vi "path array.vi"(10 "Array":string[](array[string]), 11 "file path (dialog if empty)":path=path "D:/Gantry_General/Main/ms_kao/gantry path/path data/20211103xxx.TXT") -> (3 "path array":path[](array[path]))   [LabVIEW 2016]
panel:
  out "size(s)":i32
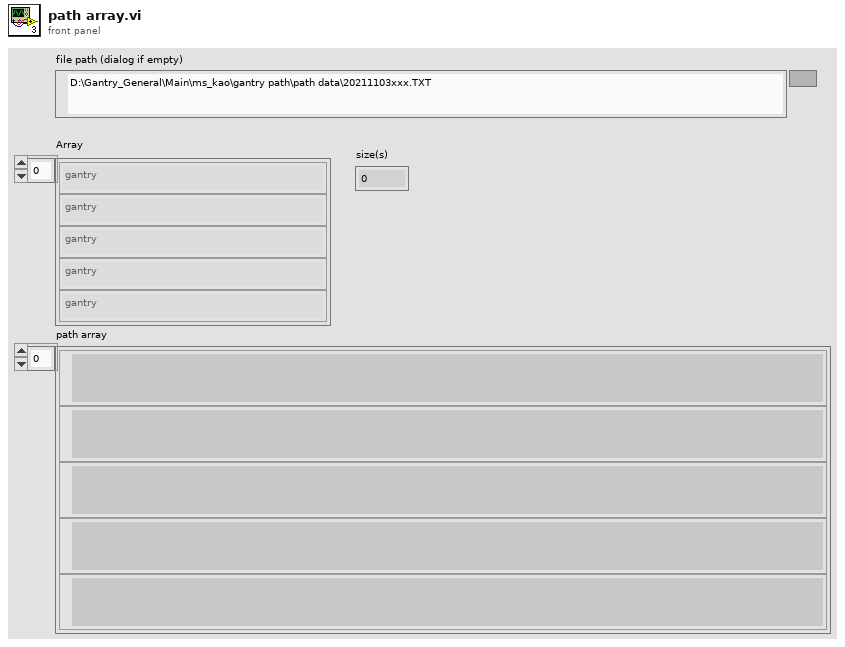
[diagram p1: front panel]
types:
  T1 = cluster{"Path":path, "folder name":string, "file name":string, "extension":string, "add time string":bool}
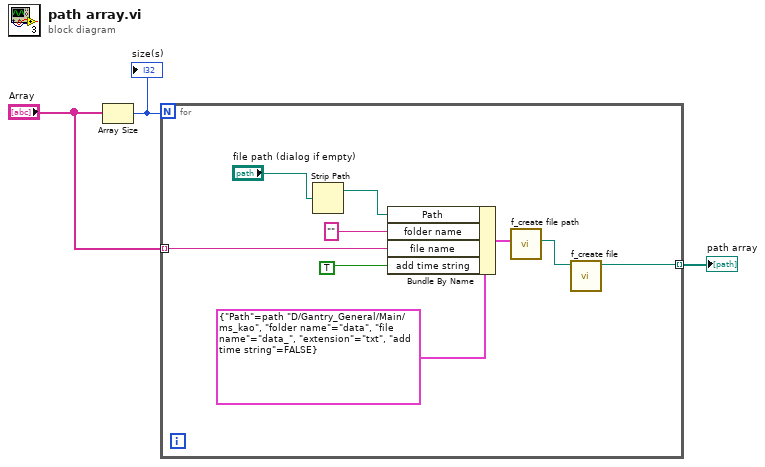
[diagram p0: block diagram]
diagram:
  n1 = Array Size(array="Array") -> (size(s)=w2:i32)
  "size(s)" <- w2
  n2 = for {
    N: w2 -> [_]
    tunnel: "Array" -> [w5] mode=indexing
    tunnel: [w4] -> w3 mode=indexing
    n3 = Strip Path(path="file path (dialog if empty)") -> (stripped path=w6:path)  [unwired: 1 out]
    n4 = Bundle By Name(cluster=T1 {"Path"=path "D:/Gantry_General/Main/ms_kao", "folder name"="data", "file name"="data_", "extension"="txt", "add time string"=FALSE} ("folder and file name Cluster"), "Path"=w6, "folder name"="", "file name"=w5, "add time string"=TRUE) -> (w11:T1)
    n5 = call "f_create file path.vi"("folder and file name Cluster"=w11) -> ("appended path"=w9:path)  [unwired: 10 in]
    n6 = call "f_create file.vi"("path"=w9) -> ("dup path"=w4:path)  [unwired: 10 in]
  }
  "path array" <- w3
